vi "Read Channel Active.vi"(8 "error in":errorcluster, 11 "Input Channels in":refnum<class "Input Channels.lvclass">) -> (0 "error out":errorcluster, 2 "Channel Active":bool, 3 "Input Channels out":refnum<class "Input Channels.lvclass">)   [LabVIEW 2020, in "Plugin.lvlib" / "Input Channels.lvclass"]
doc: "Reads channel active."
uses:
  Input Channels.lvclass
  Input Channels.lvclass/Input Channels.ctl
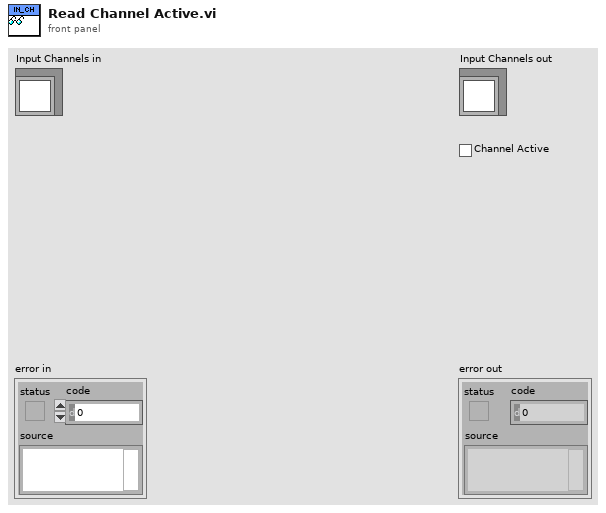
[diagram p1: front panel]
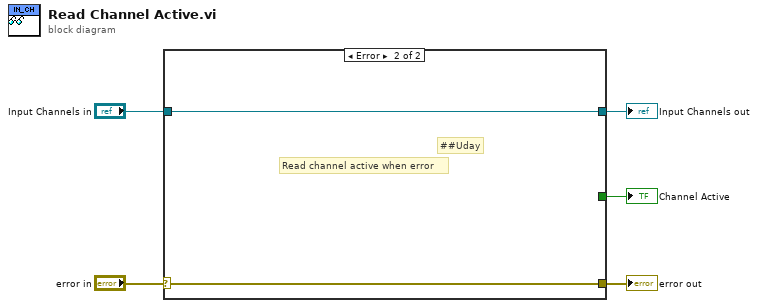
[diagram p0: block diagram]
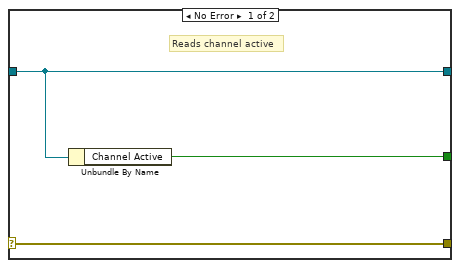
[diagram p2: hidden frame]
diagram:
  n1 = case shown="Error" "error in" {
    selector: "error in" -> [w8 w9]
    tunnel: [w8 w9] -> w4
    tunnel: [w7 w10] -> w2
    tunnel: "Input Channels in" -> [w7 w10]
    tunnel: [w6 _] -> w1
    frame No Error {
      # "Reads channel active"
      n2 = Unbundle By Name(w7) -> ("Channel Active"=w6:bool)
    }
    frame Error {
      # "##Uday"
      # "Read channel active when error"
    }
  }
  "error out" <- w4
  "Input Channels out" <- w2
  "Channel Active" <- w1
